vi "Script Msg Private Data.vi"(6 "Name Msg Refs.Private Data Cluster":refnum<vi>, 8 "error in":errorcluster, 9 "Name Msg Refs.Private Data Control":refnum<vi>, 10 "Msg Terminal Attributes":T1) -> (0 "error out":errorcluster)   [LabVIEW 2025, in "_Msg Rescript.lvlib" / "_Msg Rescript.lvclass"]
uses:
  _Msg Rescript.lvclass
  Terminal Attributes.ctl
  Attributes.ctl
  <vilib>/Utility/miscctls.llb/LVPositionTypeDef.ctl
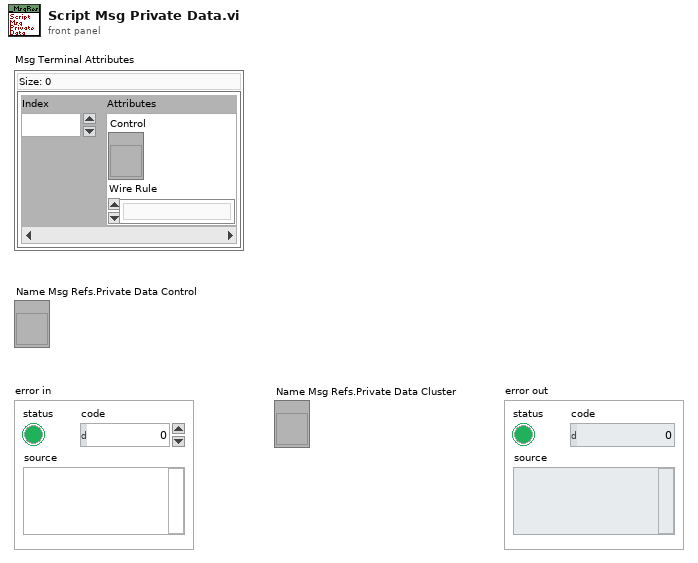
[diagram p1: front panel]
types:
  T1 = typedef "_Msg Rescript.lvlib/_Msg Rescript.lvclass/Terminal Attributes.ctl" = map{i32, T2}
  T2 = typedef "_Msg Rescript.lvlib/_Msg Rescript.lvclass/Attributes.ctl" = cluster{"Control":refnum<vi>, "Wire Rule":enum16{"Invalid Wire Rule", "Required", "Recommended", "Optional", "Dynamic Dispatch"}}
  T3 = typedef "LVPositionTypeDef.ctl" = cluster{"Left":i32, "Top":i32}
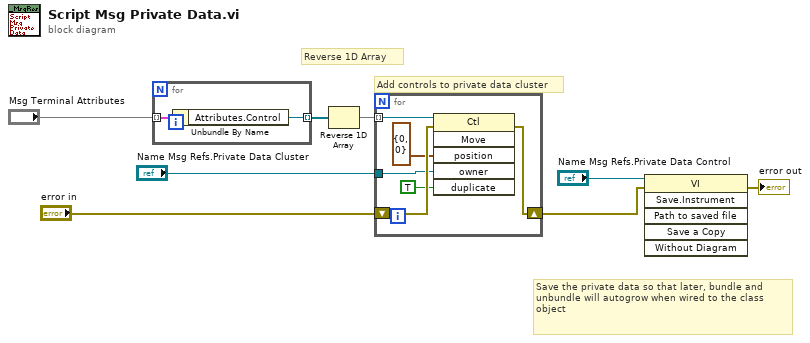
[diagram p0: block diagram]
diagram:
  # "Reverse 1D Array"
  # "Add controls to private data cluster"
  # "Save the private data so that later, bundle and unbundle will autogrow when wired to the class object"
  n1 = for {
    tunnel: "Msg Terminal Attributes" -> [w10] mode=indexing
    tunnel: [w9] -> w8 mode=indexing
    n2 = Unbundle By Name(w10) -> ("Attributes.Control"=w9:refnum<vi>)
  }
  n3 = Reverse 1D Array(array=w8) -> (reversed array=w7:refnum<vi>[])
  n4 = for {
    tunnel: "Name Msg Refs.Private Data Cluster" -> [w15]
    shift-right: [w14] -> w6
    shift-left: "error in" -> [w16]
    tunnel: w7 -> [w13] mode=indexing
    n5 = invoke class="Ctl" method="Move"(reference=w13, error in=w16, "position"=T3 {"Left"=0, "Top"=0}, "owner"=w15, "duplicate"=TRUE ("Duplicate? (F)")) -> (error out=w14:errorcluster)  [unwired: 1 in, 5 out]
  }
  n6 = invoke class="VI" method="Save.Instrument"(reference="Name Msg Refs.Private Data Control", error in=w6) -> (error out=→"error out":errorcluster)  [unwired: 4 in, 5 out]
